vi "Send Handle Vecto Message.vi"(7 "Message Priority (Normal)":T2=enum."Normal", 8 "error in (no error)":errorcluster, 10 "TcpPayload":T1, 11 "Message Enqueuer":refnum<class "Message Enqueuer.lvclass">) -> (0 "error out":errorcluster, 3 "Message Enqueuer out":refnum<class "Message Enqueuer.lvclass">)   [LabVIEW 2020, in "Volatus.lvlib" / "Handle Vecto Message Msg.lvclass"]
doc: "This VI sends the message to an actor."
uses:
  Handle Vecto Message Msg.lvclass
  <vilib>/ActorFramework/Message Enqueuer/Message Enqueuer.lvclass
  <vilib>/ActorFramework/Message Enqueuer/Message Priority.ctl
  lv-vecto/Vecto/proto/TcpPayload/Data.ctl
  C:/Program Files (x86)/National Instruments/LabVIEW 2020/vi.lib/ActorFramework/Message/Message.lvclass
  Handle Vecto Message Msg.lvclass/Handle Vecto Message Msg.ctl
  <vilib>/ActorFramework/Message Enqueuer/Message Enqueuer.lvclass/Message Enqueuer.ctl
  <vilib>/ActorFramework/Message Priority Queue/Priority Enqueue.vi
  C:/dev/lv20CE/relink/lv-volatus/Volatus/VectoMessageHandler Messages/Handle Vecto Message Msg/Handle Vecto Message Msg.lvclass
  lv-vecto/Vecto/proto/TcpPayload/TcpPayload.lvlib
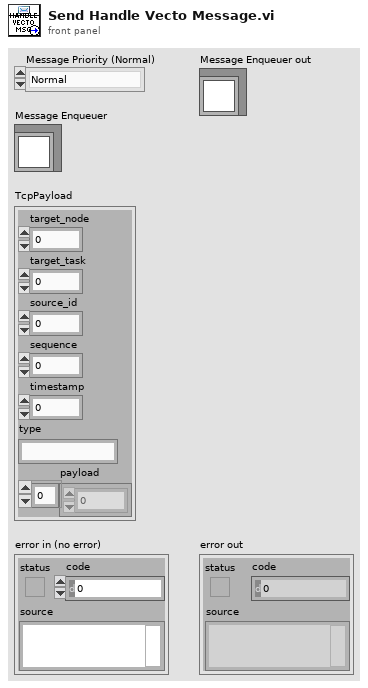
[diagram p1: front panel]
types:
  T1 = typedef "TcpPayload.lvlib/Data.ctl" = cluster{"target_node":u32, "target_task":u32, "source_id":u32, "sequence":u32, "timestamp":u64, "type":string, "payload":u8[]}
  T2 = typedef "Actor Framework.lvlib/Message Enqueuer.lvclass/Message Priority.ctl" = enum16{"Low", "Normal", "High"}
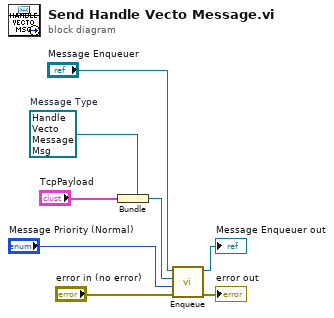
[diagram p0: block diagram]
diagram:
  w5 = refnum<class "Handle Vecto Message Msg.lvclass"> refnum  # Message Type
  n1 = Bundle(cluster=w5, "TcpPayload") -> (w4:refnum<class "Handle Vecto Message Msg.lvclass">)
  n2 = call <vilib>:"Enqueue.vi"("error in (no error)"="error in (no error)", "Message Priority (Normal)"="Message Priority (Normal)", "Message"=w4, "Message Enqueuer in"="Message Enqueuer") -> ("error out"=→"error out":errorcluster, "Message Enqueuer in"=→"Message Enqueuer out":refnum<class "Message Enqueuer.lvclass">)  [unwired: 6 in]
